vi "PolynomialFit.vi"() -> ()   [LabVIEW 2013]
panel:
  out "a2":dbl
  out "a1":dbl
  out "a0":dbl
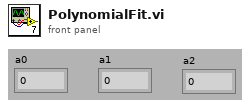
[diagram p1: front panel]
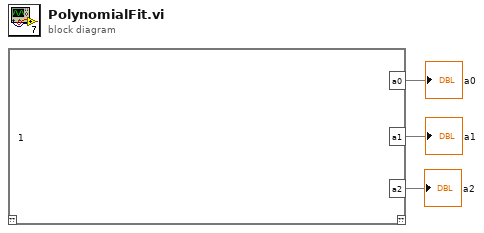
[diagram p0: block diagram]
diagram:
  n1 = mathscript code="1"() -> ("a0"=→"a0", "a1"=→"a1", "a2"=→"a2")  [unwired: 1 in, 1 out]
